vi "Write Force Setpoint.vi"(10 "Force Setpoint":dbl[unit], 11 "StartOpenLoopScan in":refnum<class "StartOpenLoopScan.lvclass">) -> (3 "StartOpenLoopScan out":refnum<class "StartOpenLoopScan.lvclass">)   [LabVIEW 2015]
uses:
  StartOpenLoopScan.lvclass
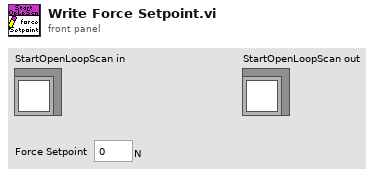
[diagram p1: front panel]
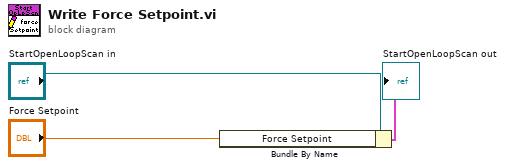
[diagram p0: block diagram]
diagram:
  n1 = Bundle By Name(cluster="StartOpenLoopScan in", "Force Setpoint"="Force Setpoint") -> (→"StartOpenLoopScan out":cluster{})
